vi "test-trapezoid-profile-timing-to-negative-goal.vi"() -> (3 "Test Passed":bool)   [LabVIEW 2019]
uses:
  <vilib>/Rock Robotics/WPI/ThirdParty/JAS_Junk/TrajLib/TRAPEZOID_PROFILE_STATE.ctl
  <vilib>/Rock Robotics/WPI/ThirdParty/JAS_Junk/TrajLib/TRAPEZOID_PROFILE.ctl
  <vilib>/Rock Robotics/WPI/ThirdParty/JAS_Junk/TrajLib/TRAPEZOID_PROFILE_CONSTRAINT.ctl
  <vilib>/Rock Robotics/WPI/ThirdParty/JAS_Junk/TrajLib/TrapProfile_Direct.vi
  <vilib>/Rock Robotics/WPI/ThirdParty/JAS_Junk/TrajLib/TrapProfile_ShouldFlipAcceleration.vi
  <vilib>/Rock Robotics/SystemInterfaces/NetworkCommunication/NetComm_UsageReport_report.vi
  <vilib>/Rock Robotics/WPI/ThirdParty/JAS_Junk/TrajLib/Util_LibraryGlobals.vi
  <vilib>/Rock Robotics/WPI/ThirdParty/JAS_Junk/TrajLib/Trajectory_Library.lvlib
panel:
  out "ApproxEquals 2":bool
  out "ApproxEquals":bool
  out "Equal":bool
  out "ActualTime":dbl
  out "PredictedTImeLeft":dbl
  out "TimeLeftGoal":dbl
  out "TimeLeftPos":dbl
  out "ReachedGoal":bool
  out "TotalTime":dbl
  out "TRAPEZOID_PROFILE":T1 {"Goal"."Velocity" format="%16_6e"; "Goal"."Position" format="%16_6e"; "Initial"."Velocity" format="%16_6e"; "Initial"."Position" format="%16_6e"; "Constraints"."MaxAcceleration" format="%16_6e"; "Constraints"."MaxVelocity" format="%16_6e"; "EndDecel" format="%16_6e"; "EndFullSpeed" format="%16_6e"; "EndAccel" format="%16_6e"}
  out "State":T3 {"Velocity" format="%16_6e"; "Position" format="%16_6e"}
  out "Waveform Chart":T4(graph)
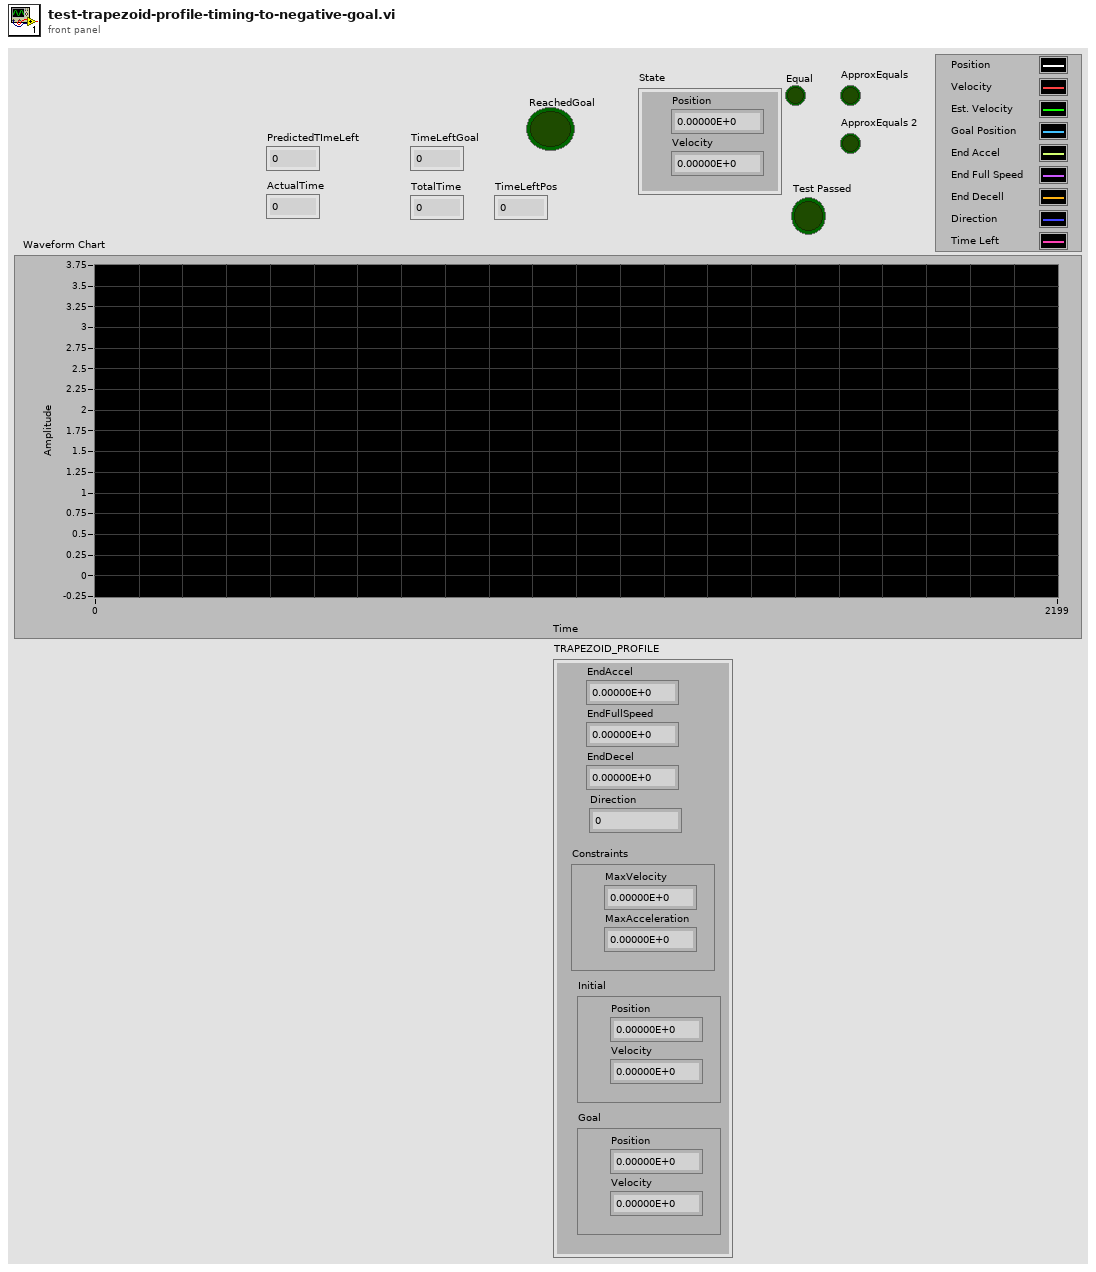
[diagram p1: front panel]
types:
  T1 = typedef "Trajectory_Library.lvlib/TRAPEZOID_PROFILE.ctl" = cluster{"EndAccel":dbl, "EndFullSpeed":dbl, "EndDecel":dbl, "Direction":i32, "Constraints":T2, "Initial":T3, "Goal":T3}
  T2 = typedef "Trajectory_Library.lvlib/TRAPEZOID_PROFILE_CONSTRAINT.ctl" = cluster{"MaxVelocity":dbl, "MaxAcceleration":dbl}
  T3 = typedef "Trajectory_Library.lvlib/TRAPEZOID_PROFILE_STATE.ctl" = cluster{"Position":dbl, "Velocity":dbl}
  T4 = cluster{"Position":dbl, "Velocity":dbl, dbl, "Position":dbl, "EndAccel":dbl, "EndFullSpeed":dbl, "EndDecel":dbl, "Direction":i32, "Position":dbl}
  T5 = cluster{"Position":dbl, "Velocity":dbl, dbl, "Position":dbl, "EndAccel":dbl, "EndFullSpeed":dbl, "EndDecel":dbl, "Direction":i32, "TimeLeft":dbl}
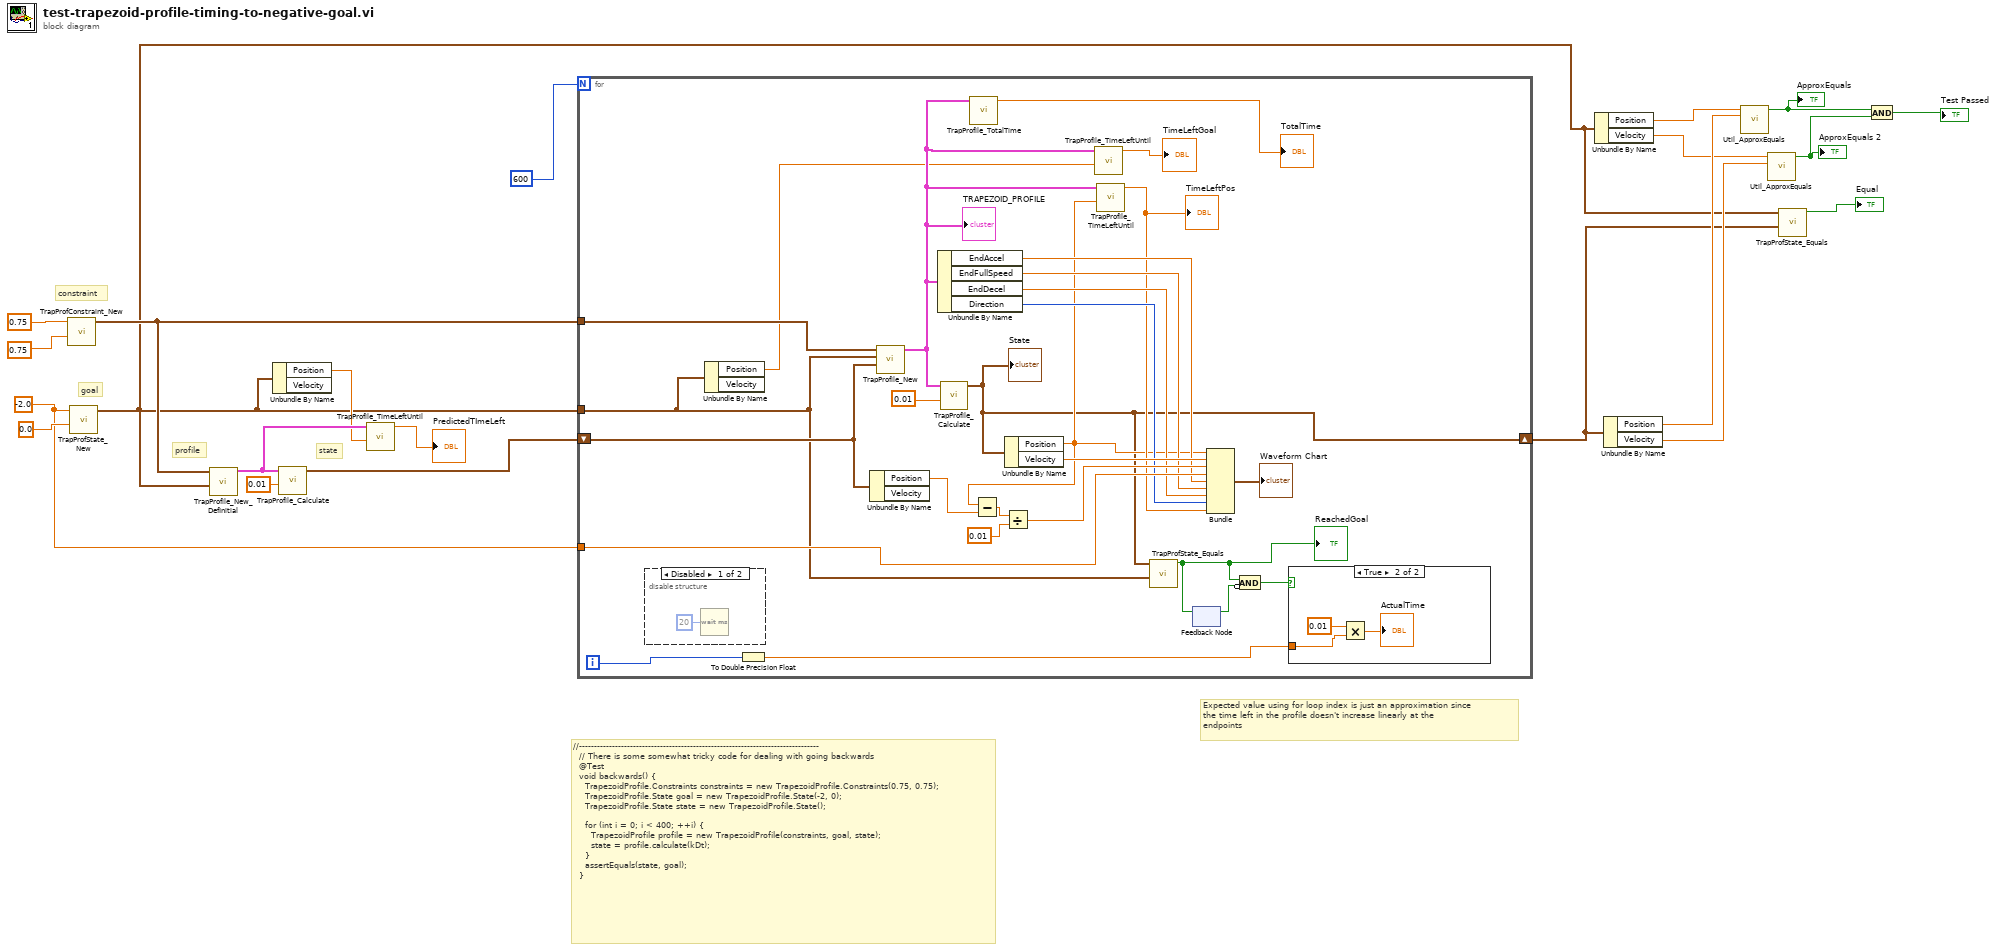
[diagram p0: block diagram]
diagram:
  w17 = -2.0 ("Position")
  # "Expected value using for loop index is just an approximation since\nthe time left in the profile doesn't increase linearly at the\nendpoints"
  # "profile"
  # "state"
  # "//--------------------------------------------------------------------------------\n  // There is some somewhat tricky code for dealing with going backwards\n  @Test\n  void backwards() {\n    TrapezoidProfile.Constraints constraints = new TrapezoidProfile.Constraints(0.75, 0.75);\n    TrapezoidProfile.State goal = new TrapezoidProfile.State(-2, 0);\n    TrapezoidProfile.State state = new TrapezoidProfile.State();\n\n    for (int i = 0; i < 400; ++i) {\n      TrapezoidProfile profile = new TrapezoidProfile(constraints, goal, state);\n      state = profile.calculate(kDt);\n    }\n    assertEquals(state, goal);\n  }"
  # "goal"
  # "constraint"
  n1 = call <vilib>:"TrapProfConstraint_New.vi"("Max Accel"=0.75, "Max Speed (M/S)"=0.75) -> ("TRAPEZOID_PROFILE_CONSTRAINT"=w16:T2)  [unwired: 9 in]
  n2 = call <vilib>:"TrapProfState_New.vi"("Velocity"=0.0, "Position"=w17) -> ("TRAPEZOID_PROFILE_STATE"=w1:T3)  [unwired: 9 in]
  n3 = call <vilib>:"TrapProfile_New_DefInitial.vi"("Goal"=w1, "Constraints"=w16) -> ("TRAPEZOID_PROFILE"=w13:T1)  [unwired: 9 in]
  n4 = Unbundle By Name(w1) -> ("Position"=w12:dbl)  [unwired: 1 out]
  n5 = call <vilib>:"TrapProfile_Calculate.vi"("Time"=0.01, "TRAPEZOID_PROFILE"=w13) -> ("State"=w14:T3)  [unwired: 9 in]
  n6 = call <vilib>:"TrapProfile_TimeLeftUntil.vi"("TargetDistance"=w12, "TRAPEZOID_PROFILE"=w13) -> ("TimeLeft"=→"PredictedTImeLeft":dbl)  [unwired: 9 in]
  n7 = for {
    N: 600 -> [_]
    shift-right: [w31] -> w2
    shift-left: w14 -> [w45]
    tunnel: w1 -> [w28]
    tunnel: w17 -> [w41]
    tunnel: w16 -> [w35]
    i -> [w23]
    n8 = disable-structure shown="Disabled" {
      frame Disabled {
        n9 = Wait (ms)(milliseconds to wait=u32 20) -> ()  [unwired: 1 out]
      }
      frame Enabled {
      }
    }
    n10 = Unbundle By Name(w28) -> ("Position"=w27:dbl)  [unwired: 1 out]
    n11 = To Double Precision Float(number=w23) -> (double precision float=w22:dbl)
    n12 = Unbundle By Name(w45) -> ("Position"=w36:dbl)  [unwired: 1 out]
    n13 = call <vilib>:"TrapProfile_New.vi"("Initial"=w45, "Goal"=w28, "Constraints"=w35) -> ("TRAPEZOID_PROFILE"=w30:T1)  [unwired: 8 in]
    "TRAPEZOID_PROFILE" <- w30
    n14 = Unbundle By Name(w30) -> ("EndAccel"=w40:dbl, "EndFullSpeed"=w39:dbl, "EndDecel"=w38:dbl, "Direction"=w37:i32)
    n15 = call <vilib>:"TrapProfile_Calculate.vi"("Time"=0.01, "TRAPEZOID_PROFILE"=w30) -> ("State"=w31:T3)  [unwired: 9 in]
    "State" <- w31
    n16 = call <vilib>:"TrapProfile_TotalTime.vi"("TRAPEZOID_PROFILE"=w30) -> ("TotalTime"=→"TotalTime":dbl)  [unwired: 10 in]
    n17 = Unbundle By Name(w31) -> ("Position"=w33:dbl, "Velocity"=w47:dbl)
    n18 = Subtract(x=w33, y=w36) -> (x-y=w44:dbl)
    n19 = Divide(x=w44, y=0.01) -> (x/y=w42:dbl)
    n20 = call <vilib>:"TrapProfile_TimeLeftUntil.vi"("TargetDistance"=w27, "TRAPEZOID_PROFILE"=w30) -> ("TimeLeft"=→"TimeLeftGoal":dbl)  [unwired: 9 in]
    n21 = call <vilib>:"TrapProfile_TimeLeftUntil.vi"("TargetDistance"=w33, "TRAPEZOID_PROFILE"=w30) -> ("TimeLeft"=w34:dbl)  [unwired: 9 in]
    "TimeLeftPos" <- w34
    n22 = call <vilib>:"TrapProfState_Equals.vi"("TRAPEZOID_PROFILE_STATE 2"=w28, "TRAPEZOID_PROFILE_STATE"=w31) -> ("Equal"=w26:bool)  [unwired: 9 in]
    "ReachedGoal" <- w26
    n23 = feedback-in #1(w26) -> ()
    n24 = feedback #1() -> (w25:bool)  [unwired: 1 in]
    n25 = Bundle("Position"=w33, "Velocity"=w47, w42, "Position"=w41, "EndAccel"=w40, "EndFullSpeed"=w39, "EndDecel"=w38, "Direction"=w37, "TimeLeft"=w34) -> (→"Waveform Chart":T5)  [unwired: 1 in]
    n26 = Compound Arithmetic op=AND(w26, invert w25) -> (w24:bool)
    n27 = case shown="True" w24 {
      tunnel: w22 -> [_ w52]
      frame False {
      }
      frame True {
        n28 = Multiply(x=0.01, y=w52) -> (x*y=→"ActualTime":dbl)
      }
    }
  }
  n29 = Unbundle By Name(w1) -> ("Position"=w10:dbl, "Velocity"=w8:dbl)
  n30 = Unbundle By Name(w2) -> ("Position"=w9:dbl, "Velocity"=w6:dbl)
  n31 = call <vilib>:"Util_ApproxEquals.vi"("Value 2"=w9, "Value 1"=w10) -> ("ApproxEquals"=w4:bool)  [unwired: 9 in]
  "ApproxEquals" <- w4
  n32 = call <vilib>:"Util_ApproxEquals.vi"("Value 2"=w6, "Value 1"=w8) -> ("ApproxEquals"=w3:bool)  [unwired: 9 in]
  "ApproxEquals 2" <- w3
  n33 = call <vilib>:"TrapProfState_Equals.vi"("TRAPEZOID_PROFILE_STATE 2"=w2, "TRAPEZOID_PROFILE_STATE"=w1) -> ("Equal"=→"Equal":bool)  [unwired: 9 in]
  n34 = And(x=w4, y=w3) -> (x .and. y?=→"Test Passed":bool)
